vi "Solve2.vi"(8 "Error In":errorcluster, 11 "object in":refnum<class "2024_1.lvclass">) -> (0 "Error Out":errorcluster, 2 "Result":u64, 3 "object out":refnum<class "2024_1.lvclass">)   [LabVIEW 2023, in "2024_1.lvclass"]
uses:
  2024_1.lvclass
  2024_1.lvclass/2024_1.ctl
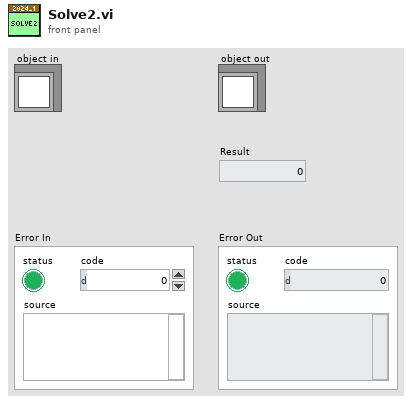
[diagram p1: front panel]
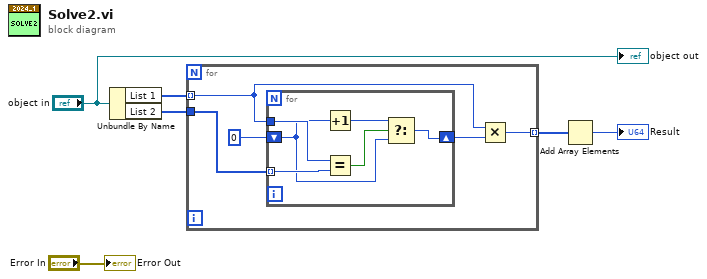
[diagram p0: block diagram]
diagram:
  n1 = Unbundle By Name("object in") -> ("List 1"=w4:i64[], "List 2"=w3:i64[])
  n2 = for {
    tunnel: w4 -> [w9] mode=indexing
    tunnel: w3 -> [w11]
    tunnel: [w7] -> w1 mode=indexing
    n3 = for {
      tunnel: w9 -> [w16]
      tunnel: w11 -> [w17] mode=indexing
      shift-right: [w13] -> w8
      shift-left: 0 -> [w14]
      n4 = Increment(x=w14) -> (x+1=w12:i32)
      n5 = Equal?(x=w16, y=w17) -> (x = y?=w15:bool)
      n6 = Select(t=w12, s=w15, f=w14) -> (s? t:f=w13:i32)
    }
    n7 = Multiply(x=w9, y=w8) -> (x*y=w7:i64)
  }
  n8 = Add Array Elements(numeric array=w1) -> (sum=→"Result":i64)
  "Error Out" <- "Error In"
  "object out" <- "object in"
